vi "Are Channels Valid.vi"(8 "error in (no error)":errorcluster, 10 "Channels In":string[](array[string]), 11 "SDF Path":path) -> (0 "error out":errorcluster, 1 "Invalid Channels Found?":bool, 2 "Invalid Channels Out":string[](array[string]), 3 "Valid Channels Out":string[](array[string]))   [LabVIEW 2015]
uses:
  NationalInstruments.VeriStand.SystemDefinitionAPI
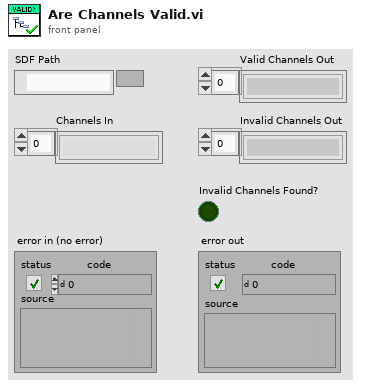
[diagram p1: front panel]
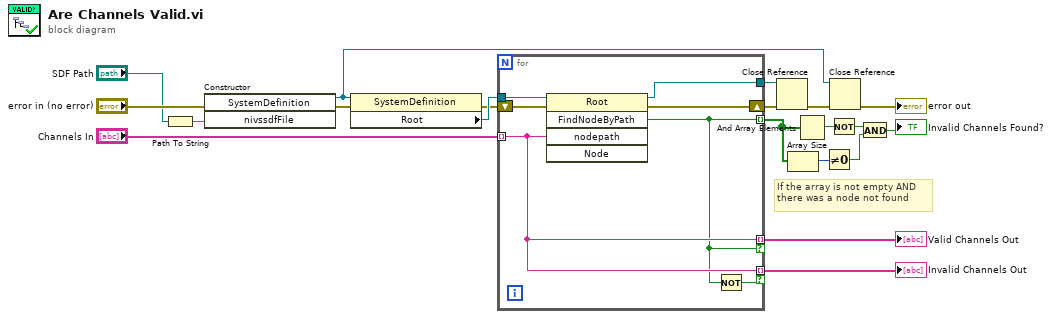
[diagram p0: block diagram]
diagram:
  # "If the array is not empty AND there was a node not found"
  n1 = Path To String(path="SDF Path") -> (string=w19:string)
  n2 = constructor class="SystemDefinition"(error in="error in (no error)", "nivssdfFile"=w19) -> (reference out=w9:refnum<k24>, error out=w16:errorcluster)  [unwired: 2 in, 2 out]
  n3 = property class="SystemDefinition"(reference=w9, error in=w16) -> (error out=w13:errorcluster, "Root"=w17:refnum<k24>)  [unwired: 1 out]
  n4 = for {
    tunnel: w17 -> [w27]
    tunnel: "Channels In" -> [w23] mode=indexing
    tunnel: [w21] -> w5 mode=indexing
    shift-right: [w26] -> w14
    shift-left: w13 -> [w25]
    tunnel: [w24] -> w11
    tunnel: [w23] -> w2 mode=indexing if=w21
    tunnel: [w23] -> w1 mode=indexing if=w22
    n5 = invoke class="Root" method="FindNodeByPath"(reference=w27, error in=w25, "nodepath"=w23) -> (reference out=w24:refnum<k24>, error out=w26:errorcluster, "FindNodeByPath"=w21:bool)  [unwired: 2 in, 2 out]
    n6 = Not(x=w21) -> (.not. x?=w22:bool)
  }
  "Valid Channels Out" <- w2
  "Invalid Channels Out" <- w1
  n7 = Close Reference(reference=w11, error in (no error)=w14) -> (error out=w12:errorcluster)
  n8 = Array Size(array=w5) -> (size(s)=w4:i32)
  n9 = And Array Elements(Boolean array=w5) -> (logical AND=w8:bool)
  n10 = Not Equal To 0?(x=w4) -> (x != 0?=w3:bool)
  n11 = Not(x=w8) -> (.not. x?=w7:bool)
  n12 = Close Reference(reference=w9, error in (no error)=w12) -> (error out=→"error out":errorcluster)
  n13 = And(x=w7, y=w3) -> (x .and. y?=→"Invalid Channels Found?":bool)
